vi "MessageAI_State.vi"(8 "Port: 2":u16=20011, 9 "Port:":u16=20011, 10 "SSL Vision Address:":string="127.0.0.1", 11 "IA state":T1={"our_robots"=[], "enemy_robots"=[], "balls"=[], "geometry"={"line_width"=0, "field_length"=0, "field_width"=0, "boundary_width"=0, "referee_width"=0, "goal_width"=0, "goal_depth"=0, "goal_wall_width"=0, "center_circle_radius"=0, "defense_radius"=0, "defense_stretch"=0, "free_kick_from_defense_dist"=0, "penalty_spot_from_field_line_dist"=0, "penalty_line_from_spot_dist"=0}, "IA Judge"={"stage"="", "command"="", "our_goalie_id"=0.0, "enemy_goalie_id"=0.0, "command enum"=enum."Halt", "Time"=enum."Azul"}, "Received Timestamp"=timestamp(0 s since 1904-01-01), "Events"={"Touch"=FALSE, "Ball out"=FALSE, "id touch"=0.0, "Ball out of \nVision"=FALSE, "Ball inside \nGoalie area"=FALSE, "Robot not responding"=FALSE, "Robots responding status"=[1.0, 1.0, 1.0, 1.0, 1.0, 1.0], "Enemy Ball \nPossession"=FALSE, "Pass State"=FALSE, "id end of pass"=0.0, "Kick"=FALSE, "Id ini Possession"=0.0, "Ball Possesion"=FALSE, "Id Possesion"=0.0, "Direct Kick"=FALSE, "2nd Strk Ativo"=FALSE}}) -> ()   [LabVIEW 2023]
uses:
  Vision_class/Old vision/SSL Detection Frame Simple Estimator Cameras VelCmd Folder/Core/AI Input.ctl
  Vision_class/Old vision/Controls/AI Robot.ctl
  Vision_class/Old vision/Controls/Functions Enum.ctl
  Vision_class/Old vision/Controls/AttackerStates.ctl
  Vision_class/Old vision/Controls/PathDests.ctl
  Vision_class/Old vision/Controls/PathDest.ctl
  Game_class/Navigation/VSSNavigation/VSSAttackerStates.ctl
  Vision_class/Old vision/SSL Detection Frame Simple Estimator Cameras VelCmd Folder/Core/AI Ball.ctl
  Vision_class/Old vision/SSL Detection Frame Simple Estimator Cameras VelCmd Folder/Core/Field Size.ctl
  Vision_class/Old vision/SSL Detection Frame Simple Estimator Cameras VelCmd Folder/Core/AI Judge.ctl
  Intel/Command Enum.ctl
  Vision_class/Old vision/SSL Detection Frame Simple Estimator Cameras VelCmd Folder/Util/Events/Events.ctl
panel:
  out "Array 2":u8[](array[numeric])
  out "error out 2":errorcluster
  out "Array":u8[](array[numeric]) format="%02x"
  out "error out":errorcluster
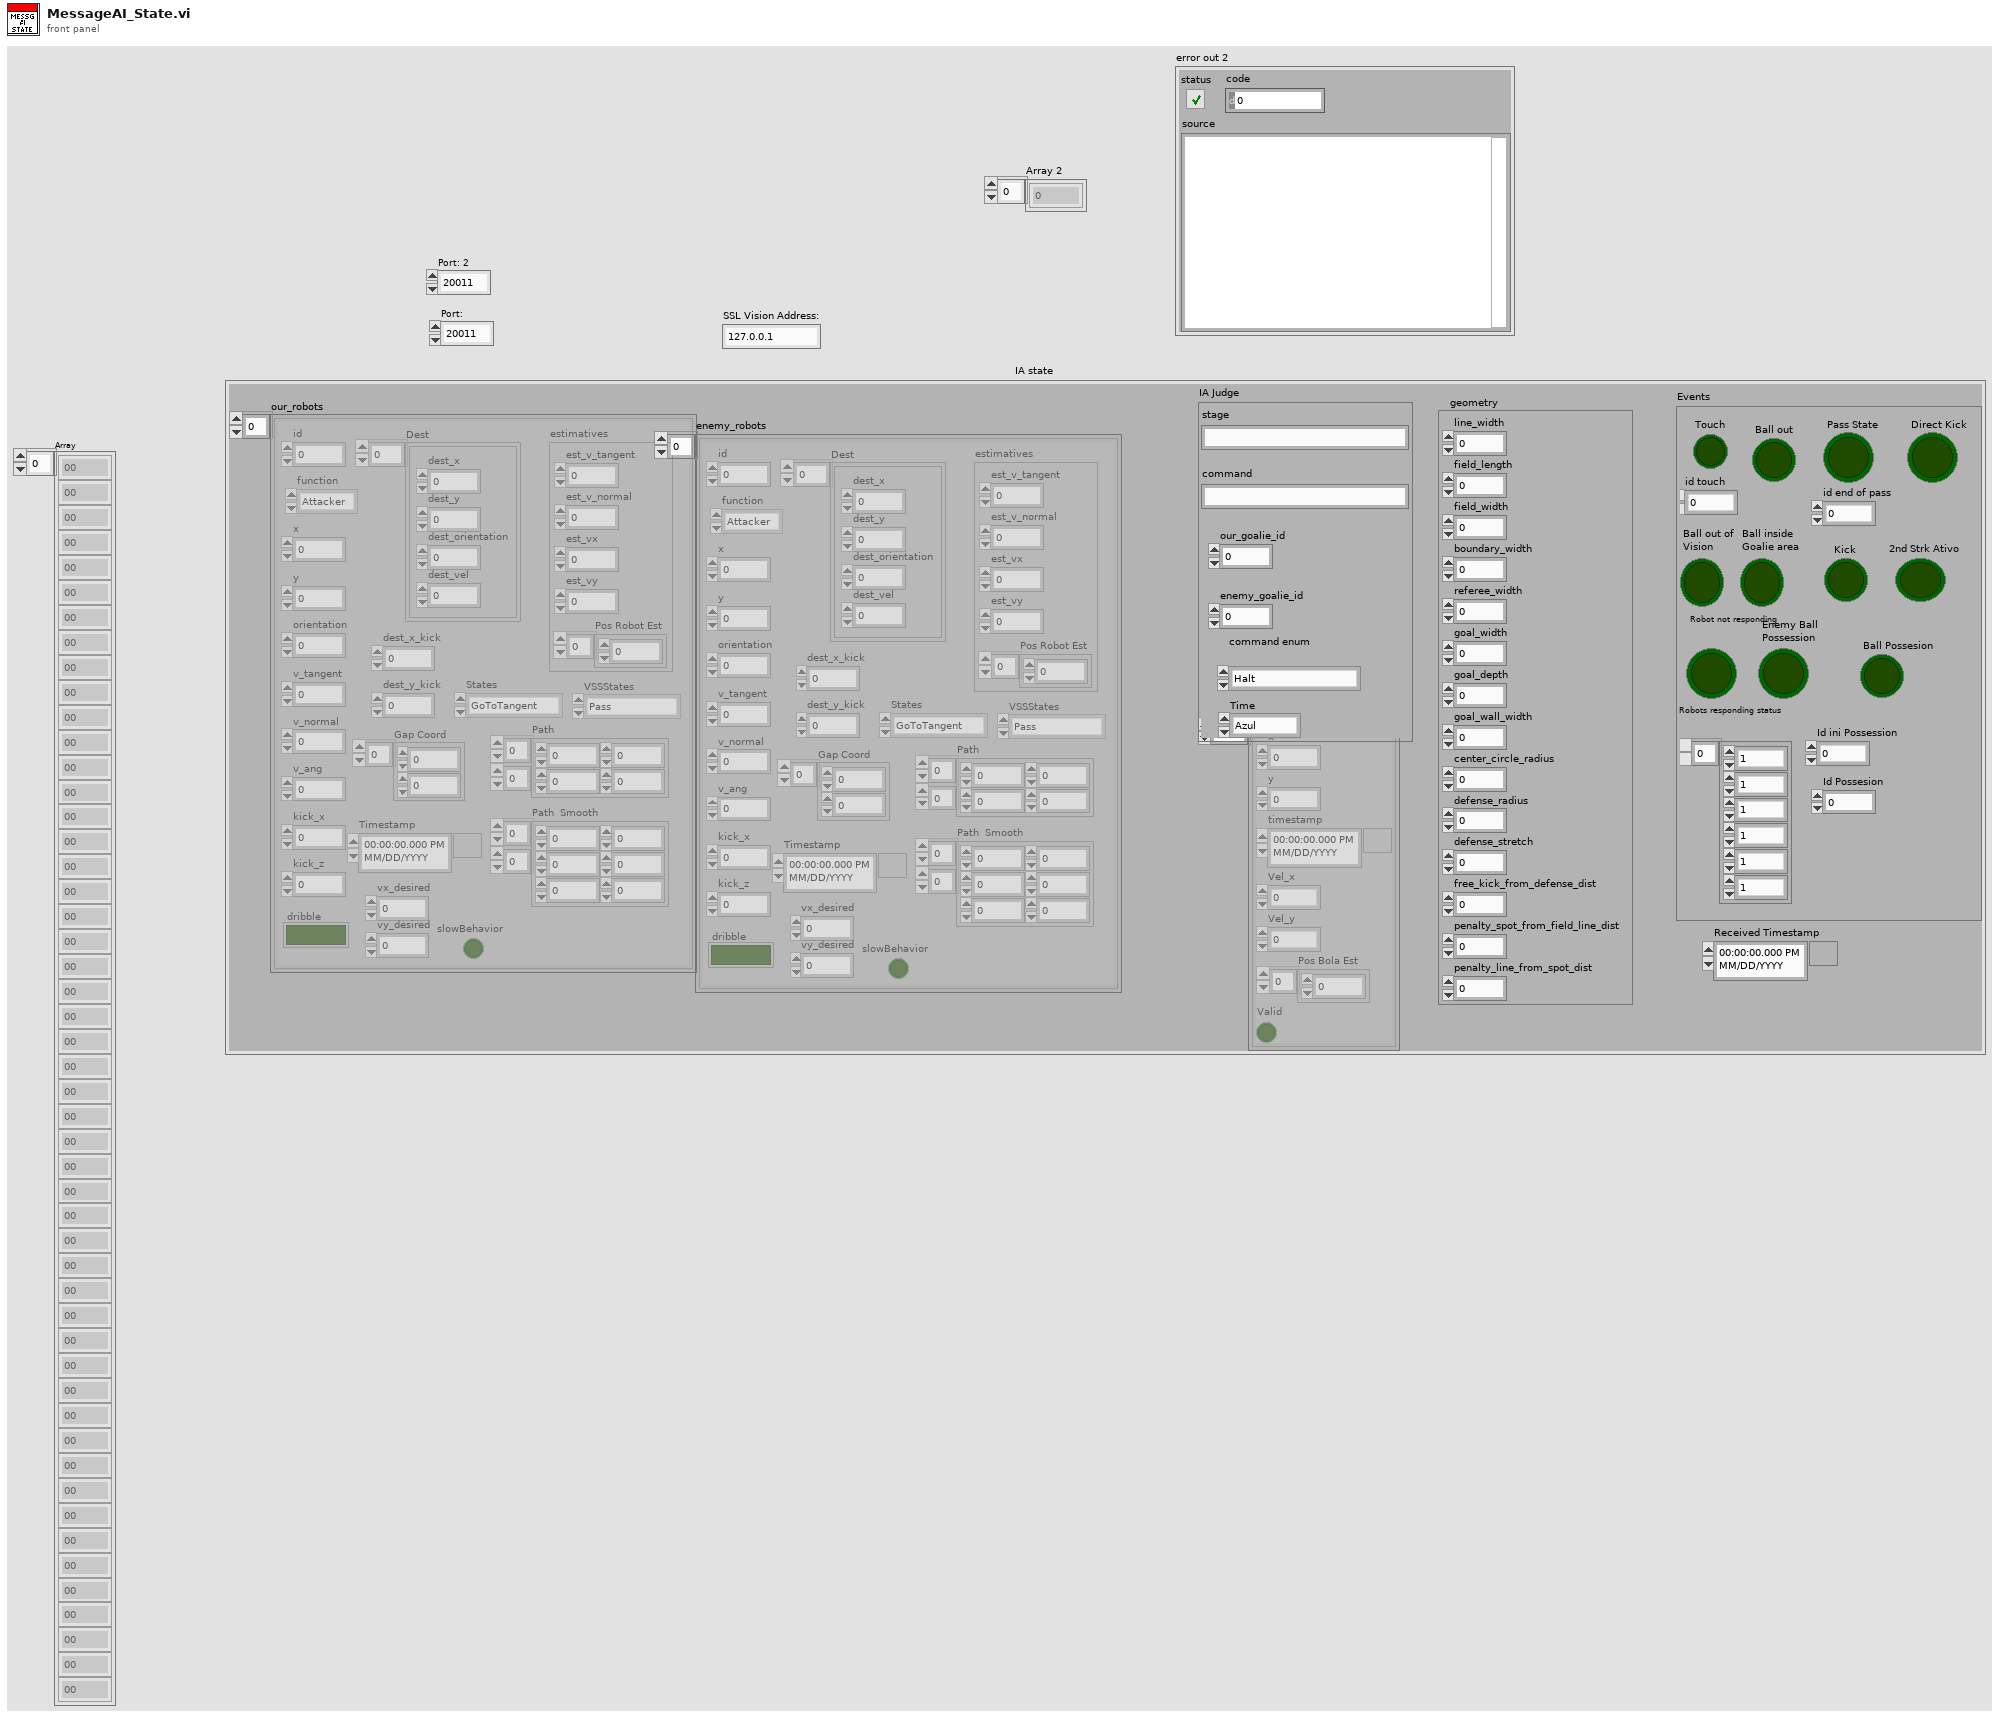
[diagram p1: front panel]
types:
  T1 = typedef "AI Input.ctl" = cluster{"our_robots":T2[], "enemy_robots":T2[], "balls":T8[], "geometry":T9, "IA Judge":T10, "Received Timestamp":timestamp, "Events":T12}
  T2 = typedef "AI Robot.ctl" = cluster{"id":u32, "function":T3, "x":dbl, "y":dbl, "orientation":dbl, "v_tangent":dbl, "v_normal":dbl, "v_ang":dbl, "kick_x":dbl, "kick_z":dbl, "dribble":bool, "Timestamp":timestamp, "estimatives":cluster{"est_v_tangent":dbl, "est_v_normal":dbl, "est_vx":dbl, "est_vy":dbl, "Pos Robot Est":dbl[]}, "dest_x_kick":dbl, "dest_y_kick":dbl, "Gap Coord":dbl[], "States":T4, "Path ":dbl[][], "Path  Smooth":dbl[][], "Dest":T5, "vx_desired":dbl, "vy_desired":dbl, "slowBehavior":bool, "VSSStates":T7}
  T3 = typedef "Functions Enum.ctl" = enum16{"2nd Striker", "Attacker", "Goalie", "Defender", "Striker", "Goto 0", "Dummy", "Kicker", "ZigZag 0", "ZigZag 1", "ZigZag 2", "ZigZag 3", "ZigZag 4", "ZigZag 5", "ZigZag 6", "ZigZag 7", "ZigZag 8", ""}
  T4 = typedef "AttackerStates.ctl" = enum16{"Pass", "GoToTangent", "BallGetting", "GoToKick", ""}
  T5 = typedef "PathDests.ctl" = T6[]
  T6 = typedef "PathDest.ctl" = cluster{"dest_x":dbl, "dest_y":dbl, "dest_orientation":dbl, "dest_vel":dbl}
  T7 = typedef "VSSAttackerStates.ctl" = enum16{"Pass", "GoToTangent", "BallGetting", "GoToKick", "Rotate anti-clockwise", "Rotate Clockwise", ""}
  T8 = typedef "AI Ball.ctl" = cluster{"x":dbl, "y":dbl, "timestamp":timestamp, "Vel_x":dbl, "Vel_y":dbl, "Pos Bola Est":dbl[], "Valid":bool}
  T9 = typedef "Field Size.ctl" = cluster{"line_width":u32, "field_length":u32, "field_width":u32, "boundary_width":u32, "referee_width":u32, "goal_width":u32, "goal_depth":u32, "goal_wall_width":u32, "center_circle_radius":u32, "defense_radius":u32, "defense_stretch":u32, "free_kick_from_defense_dist":u32, "penalty_spot_from_field_line_dist":u32, "penalty_line_from_spot_dist":u32}
  T10 = typedef "AI Judge.ctl" = cluster{"stage":string, "command":string, "our_goalie_id":dbl, "enemy_goalie_id":dbl, "command enum":T11, "Time":enum16{"Azul", "Amarelo"}}
  T11 = typedef "Command Enum.ctl" = enum16{"Halt", "Stop", "Force Start", "PKA Normal Start", "Prepare Kickoff Ally", "PKE Normal Start", "Prepare Kickoff Enemy", "Prepare Penalty Ally", "PPA Normal Start", "Prepare Penalty Enemy", "PPE Normal Start", "Direct Free Enemy", "Direct Free Ally", "Indirect Free Enemy", "Indirect Free Ally", "Timeout Enemy", "Timeout Ally", "Goal Enemy", "Goal Ally", "Ball Placement Enemy", "Ball Placement Ally", "Normal Half Time", "Extra Time Break", "Extra Half Time", "None", "Post Game"}
  T12 = typedef "Events.ctl" = cluster{"Touch":bool, "Ball out":bool, "id touch":dbl, "Ball out of \nVision":bool, "Ball inside \nGoalie area":bool, "Robot not responding":bool, "Robots responding status":dbl[], "Enemy Ball \nPossession":bool, "Pass State":bool, "id end of pass":dbl, "Kick":bool, "Id ini Possession":dbl, "Ball Possesion":bool, "Id Possesion":dbl, "Direct Kick":bool, "2nd Strk Ativo":bool}
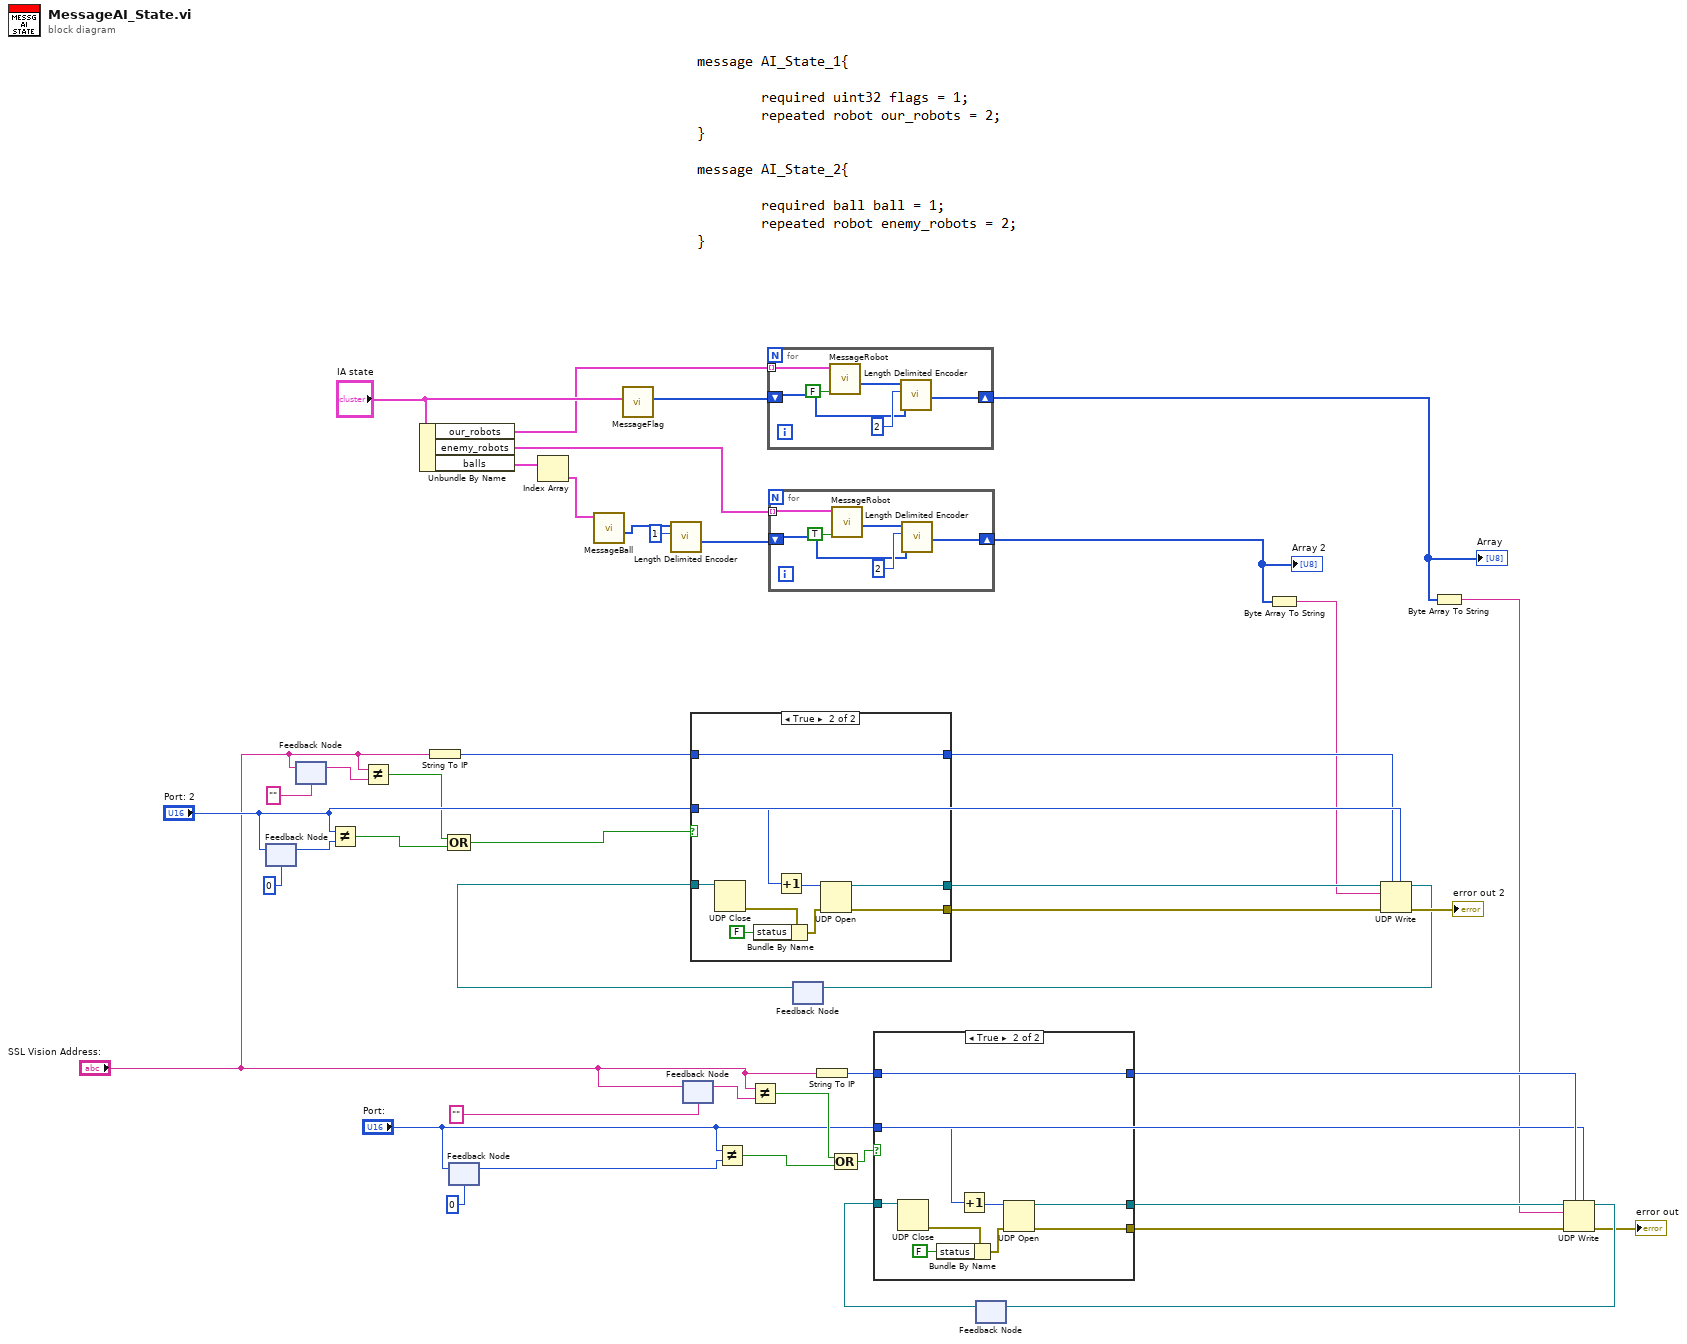
[diagram p0: block diagram]
diagram:
  n1 = feedback #1(u16 0 ("Port:")) -> (w23:u16)
  n2 = feedback-in #1("Port: 2") -> ()
  n3 = feedback #2("" ("SSL Vision Address:")) -> (w21:string)
  n4 = feedback-in #2("SSL Vision Address:") -> ()
  n5 = Not Equal?(x="Port: 2", y=w23) -> (x != y?=w19:bool)
  n6 = Not Equal?(x="SSL Vision Address:", y=w21) -> (x != y?=w20:bool)
  n7 = Unbundle By Name("IA state") -> ("our_robots"=w26:T2[], "enemy_robots"=w6:T2[], "balls"=w5:T8[])
  n8 = String To IP(1:"SSL Vision Address:") -> (0:w11:u32)
  n9 = Compound Arithmetic op=OR(w20, w19) -> (w18:bool)
  n10 = feedback #3(u16 0 ("Port:")) -> (w31:u16)
  n11 = feedback-in #3("Port:") -> ()
  n12 = Index Array(array=w5) -> (element=w4:T8)  [unwired: 1 in]
  n13 = call "MessageBall.vi"("ball"=w4) -> ("Array"=w3:u8[])  [unwired: 10 in]
  n14 = call "MessageFlag.vi"("input cluster"="IA state") -> ("Array"=w28:u8[])  [unwired: 10 in]
  n15 = call "Length Delimited Encoder.vi"("Key"=u32 1, "Array In 2"=w3) -> ("Array"=w2:u8[])  [unwired: 9 in]
  n16 = feedback #4("" ("SSL Vision Address:")) -> (w33:string)
  n17 = feedback-in #4("SSL Vision Address:") -> ()
  n18 = Not Equal?(x="Port:", y=w31) -> (x != y?=w35:bool)
  n19 = Not Equal?(x="SSL Vision Address:", y=w33) -> (x != y?=w34:bool)
  n20 = for {
    shift-right: [w50] -> w25
    shift-left: w28 -> [w48]
    tunnel: w26 -> [w47] mode=indexing
    n21 = call "MessageRobot.vi"("Enemy Robots?"=FALSE, "Robot"=w47) -> ("Array"=w46:u8[])  [unwired: 9 in]
    n22 = call "Length Delimited Encoder.vi"("Array In"=w48, "Key"=u32 2, "Array In 2"=w46) -> ("Array"=w50:u8[])  [unwired: 8 in]
  }
  "Array" <- w25
  n23 = for {
    shift-right: [w56] -> w9
    shift-left: w2 -> [w54]
    tunnel: w6 -> [w53] mode=indexing
    n24 = call "MessageRobot.vi"("Enemy Robots?"=TRUE, "Robot"=w53) -> ("Array"=w52:u8[])  [unwired: 9 in]
    n25 = call "Length Delimited Encoder.vi"("Array In"=w54, "Key"=u32 2, "Array In 2"=w52) -> ("Array"=w56:u8[])  [unwired: 8 in]
  }
  "Array 2" <- w9
  n26 = feedback #5() -> (w16:refnum<k16>)  [unwired: 1 in]
  n27 = case shown="True" w18 {
    tunnel: [_ w67] -> w24
    tunnel: [w58 w65] -> w15
    tunnel: "Port: 2" -> [_ w64]
    tunnel: w11 -> [w57 w62]
    tunnel: w16 -> [w58 w63]
    tunnel: [w57 w62] -> w10
    frame False {
    }
    frame True {
      n28 = UDP Close(connection ID=w63) -> (error out=w61:errorcluster)  [unwired: 1 in, 1 out]
      n29 = Bundle By Name(cluster=w61, "status"=FALSE) -> (w60:errorcluster)
      n30 = Increment(x=w64) -> (x+1=w66:u16)
      n31 = UDP Open(8:w60, 11:w66) -> (port=w65:refnum<k16>, 0:w67:errorcluster)  [unwired: 3 in, 1 out]
    }
  }
  n32 = String To IP(1:"SSL Vision Address:") -> (0:w43:u32)
  n33 = Compound Arithmetic op=OR(w34, w35) -> (w36:bool)
  n34 = feedback #6() -> (w38:refnum<k16>)  [unwired: 1 in]
  n35 = case shown="True" w36 {
    tunnel: [_ w78] -> w30
    tunnel: [w69 w76] -> w39
    tunnel: "Port:" -> [_ w75]
    tunnel: w43 -> [w68 w73]
    tunnel: w38 -> [w69 w74]
    tunnel: [w68 w73] -> w44
    frame False {
    }
    frame True {
      n36 = UDP Close(connection ID=w74) -> (error out=w72:errorcluster)  [unwired: 1 in, 1 out]
      n37 = Bundle By Name(cluster=w72, "status"=FALSE) -> (w71:errorcluster)
      n38 = Increment(x=w75) -> (x+1=w77:u16)
      n39 = UDP Open(8:w71, 11:w77) -> (port=w76:refnum<k16>, 0:w78:errorcluster)  [unwired: 3 in, 1 out]
    }
  }
  n40 = Byte Array To String(unsigned byte array=w9) -> (string=w8:string)
  n41 = UDP Write(address=w10, port or service name="Port: 2", connection ID=w15, data in=w8, 8:w24) -> (error out=→"error out 2":errorcluster, 3:w14:refnum<k16>)  [unwired: 1 in]
  n42 = feedback-in #5(w14) -> ()
  n43 = Byte Array To String(unsigned byte array=w25) -> (string=w29:string)
  n44 = UDP Write(address=w44, port or service name="Port:", connection ID=w39, data in=w29, 8:w30) -> (error out=→"error out":errorcluster, 3:w40:refnum<k16>)  [unwired: 1 in]
  n45 = feedback-in #6(w40) -> ()
